vi "DDVL Size and Run All.vi"(0 "Cluster Refs":refnum<vi>[](array[refnum]), 2 "Initial Top Position":i32, 7 "Subpanel Refs":refnum<vi>[](array[refnum]), 11 "VI Path/Ref":T1(array[cluster])) -> (4 "Cluster Refs Dup":refnum<vi>[](array[refnum]), 15 "VI Path/Ref Out":T1(array[cluster]))   [LabVIEW 2020]
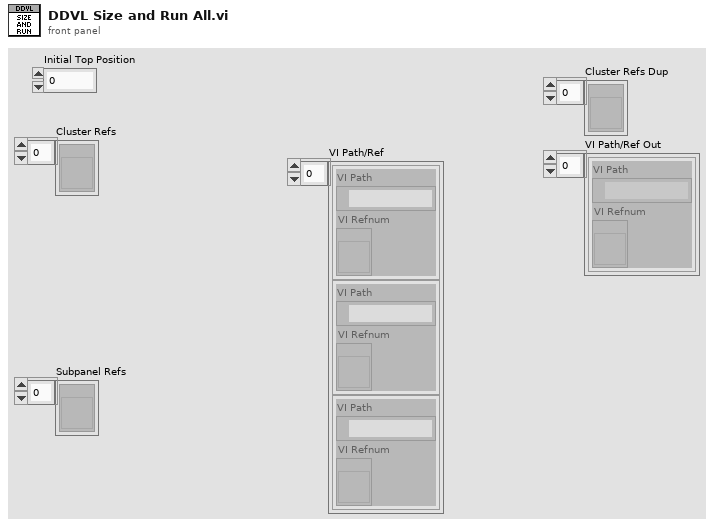
[diagram p1: front panel]
types:
  T1 = cluster{"VI Path":path, "VI Refnum":refnum<vi>}[]
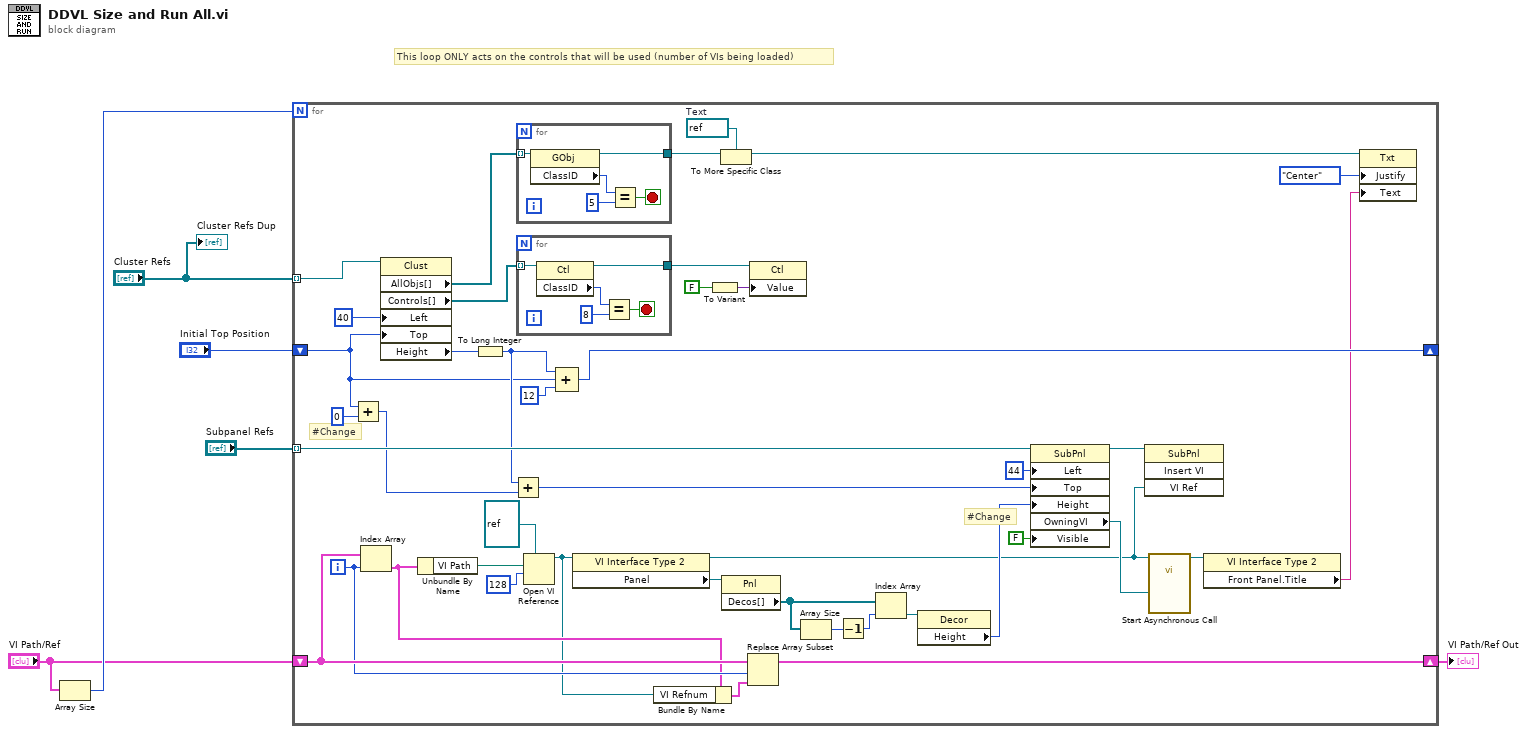
[diagram p0: block diagram]
diagram:
  # "This loop ONLY acts on the controls that will be used (number of VIs being loaded)"
  n1 = Array Size(array="VI Path/Ref") -> (size(s)=w3:i32)
  n2 = for {
    N: w3 -> [_]
    tunnel: "Cluster Refs" -> [w47] mode=indexing
    shift-right: [w46] -> _
    shift-left: "Initial Top Position" -> [w39]
    tunnel: "Subpanel Refs" -> [w44] mode=indexing
    shift-right: [w14] -> w1
    shift-left: "VI Path/Ref" -> [w16]
    i -> [w15]
    w26 = refnum<vi> refnum  # Text
    # "#Change"
    # "#Change"
    n3 = Add(x=w39, y=0) -> (x+y=w38:i32)
    n4 = Index Array(array=w16, index=w15) -> (element=w13:cluster{"VI Path":path, "VI Refnum":refnum<vi>})
    n5 = property class="Clust"(reference=w47, "Left"=40 ("Position:Left"), "Top"=w39) -> ("AllObjs[]"=w28:refnum<vi>[], "Controls[]"=w32:refnum<vi>[], "Height"=w42:u32)  [unwired: 1 in, 2 out]
    n6 = Unbundle By Name(w13) -> ("VI Path"=w12:path)
    n7 = To Long Integer(number=w42) -> (32bit integer=w41:i32)
    n8 = Add(x=w41, y=w38) -> (x+y=w40:i32)
    n9 = for {
      tunnel: w28 -> [w53] mode=indexing
      tunnel: [w50] -> w27
      stop <- w49 stop-if-true
      n10 = property class="GObj"(reference=w53) -> (reference out=w50:refnum<vi>, "ClassID"=w52:u32)  [unwired: 1 in, 1 out]
      n11 = Equal?(x=w52, y=u32 5) -> (x = y?=w49:bool)
    }
    n12 = for {
      tunnel: w32 -> [w58] mode=indexing
      tunnel: [w55] -> w31
      stop <- w54 stop-if-true
      n13 = property class="Ctl"(reference=w58) -> (reference out=w55:refnum<vi>, "ClassID"=w57:u32)  [unwired: 1 in, 1 out]
      n14 = Equal?(x=w57, y=u32 8) -> (x = y?=w54:bool)
    }
    n15 = Open VI Reference(type specifier VI Refnum (for type only)=refnum<vi> refnum, vi path=w12, options=128) -> (vi reference=w10:refnum<vi>)  [unwired: 3 in, 1 out]
    n16 = Compound Arithmetic op=ADD(w41, w39, 12 ("value")) -> (w46:i32)
    n17 = property class="VI Interface Type 2"(reference=w10) -> (reference out=w18:refnum<vi>, "Panel"=w35:refnum<vi>)  [unwired: 1 in, 1 out]
    n18 = Bundle By Name(cluster=w13, "VI Refnum"=w10) -> (w11:cluster{"VI Path":path, "VI Refnum":refnum<vi>})
    n19 = To Variant(anything=FALSE) -> (Variant=w29:variant)
    n20 = To More Specific Class(target class=w26, reference=w27) -> (specific class reference=w25:refnum<vi>)  [unwired: 1 in, 1 out]
    n21 = property class="Pnl"(reference=w35) -> ("Decos[]"=w9:refnum<vi>[])  [unwired: 1 in, 2 out]
    n22 = Replace Array Subset(array=w16, new element=w11, index=w15) -> (w14:T1)
    n23 = property class="Ctl"(reference=w31, "Value"=w29) -> ()  [unwired: 1 in, 2 out]
    n24 = Array Size(array=w9) -> (size(s)=w8:i32)
    n25 = Decrement(x=w8) -> (x-1=w7:i32)
    n26 = Index Array(array=w9, index=w7) -> (element=w34:refnum<vi>)
    n27 = property class="Decor"(reference=w34) -> ("Height"=w33:u32)  [unwired: 1 in, 2 out]
    n28 = property class="SubPnl"(reference=w44, "Left"=44 ("Position:Left"), "Top"=w40, "Height"=w33, "Visible"=FALSE) -> (reference out=w36:refnum<vi>, "OwningVI"=w22:refnum<vi>)  [unwired: 1 in, 1 out]
    n29 = invoke class="SubPnl" method="Insert VI"(reference=w36, "VI Ref"=w18) -> ()  [unwired: 2 in, 4 out]
    n30 = call-by-ref "Start Asynchronous Call"(reference=w18, "Calling VI Ref"=w22) -> (reference out=w17:refnum<vi>)  [unwired: 16 in, 1 out]
    n31 = property class="VI Interface Type 2"(reference=w17) -> ("Front Panel.Title"=w23:string)  [unwired: 1 in, 2 out]
    n32 = property class="Txt"(reference=w25, "Justify"=enum16{"Left", "Center", "Right"}."Center" ("Justification"), "Text"=w23) -> ()  [unwired: 1 in, 2 out]
  }
  "VI Path/Ref Out" <- w1
  "Cluster Refs Dup" <- "Cluster Refs"
